vi "Save LV Class For Previous Version.vi"(8 "Error In":errorcluster, 9 "LabVIEW Version":T1, 10 "Save Path":path, 11 "Class Path":path) -> (0 "Error Out":errorcluster, 2 "Warnings":string)   [LabVIEW 2011, in "LMH-Toolbox.lvlib" / "LMH-VITools.lvlib"]
uses:
  LMH-VITools.lvlib
  Type Defs/LabVIEW Version.ctl
  LMH-Toolbox.lvlib
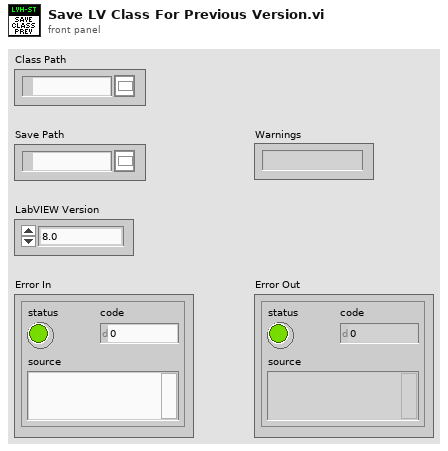
[diagram p1: front panel]
types:
  T1 = typedef "LMH-Toolbox.lvlib/LabVIEW Version.ctl" = enum16{"8.0", "8.2", "8.6", "9.0", "10.0", "11.0", "12.0", "13.0"}
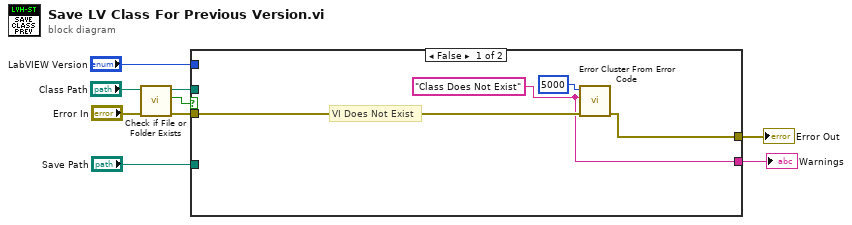
[diagram p0: block diagram]
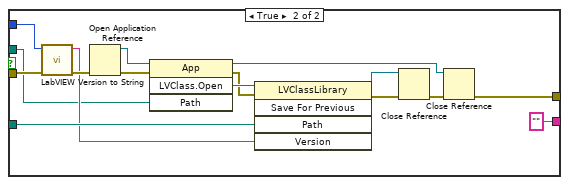
[diagram p2: hidden frame]
diagram:
  n1 = call <vilib>:"Check if File or Folder Exists.vi"("error in (no error)"="Error In", "path"="Class Path") -> ("error out"=w5:errorcluster, "file or folder exists?"=w7:bool, "dup path"=w6:path)  [unwired: 7 in]
  n2 = case shown="False" w7 {
    tunnel: w6 -> [_ w15]
    tunnel: w5 -> [w12 w28]
    tunnel: "Save Path" -> [_ w17]
    tunnel: [w13 w18] -> w3
    tunnel: [w10 "" ("error message (\"\")")] -> w2
    tunnel: "LabVIEW Version" -> [_ w29]
    frame False {
      w10 = "Class Does Not Exist" ("error message (\"\")")
      # "VI Does Not Exist"
      n3 = call <vilib>:"Error Cluster From Error Code.vi"("error in (no error)"=w12, "error message (\"\")"=w10, "error code (0)"=5000) -> ("error out"=w13:errorcluster)  [unwired: 6 in]
    }
    frame True {
      n4 = call "LabVIEW Version to String.vi"("Error In"=w28, "LabVIEW Version"=w29) -> ("Error Out"=w19:errorcluster, "LabVIEW Version"=w16:string)  [unwired: 8 in]
      n5 = Open Application Reference(8:w19) -> (0:w27:errorcluster, 3:w26:refnum<vi>)  [unwired: 3 in]
      n6 = invoke class="App" method="LVClass.Open"(reference=w26, error in=w27, "Path"=w15) -> (reference out=w20:refnum<vi>, error out=w24:errorcluster, "LVClass.Open"=w25:refnum<vi>)  [unwired: 1 in, 1 out]
      n7 = invoke class="LVClassLibrary" method="Save For Previous"(reference=w25, error in=w24, "Path"=w17, "Version"=w16) -> (reference out=w22:refnum<vi>, error out=w23:errorcluster)  [unwired: 1 in, 3 out]
      n8 = Close Reference(reference=w22, error in (no error)=w23) -> (error out=w21:errorcluster)
      n9 = Close Reference(reference=w20, error in (no error)=w21) -> (error out=w18:errorcluster)
    }
  }
  "Error Out" <- w3
  "Warnings" <- w2
